vi "rs3 configure all 2.vi"(5 "Sensor in":u64, 11 "error in (no error)":errorcluster) -> (4 "config error":string, 6 "All Available streams":T1(array[cluster]), 8 "Sensor out":u64, 15 "error out":errorcluster)   [LabVIEW 2017, in "libRealSense3.lvlib"]
doc: "This VI configures the CAMERA-SENSOR to stream a specific set of 2 PROFILES.\n\nSteam selection: \nDepth+Left Color, \nUnrectified Left + Right (The raw input images)\nRectified Left + Right\n\nThe output array of STREAM PROFILE HANDLES is used to START the streams.\n\nThis VI also returns the BASELINE of the stereo module."
uses:
  libRealSense3.lvlib
panel:
  # "RS3 Configure All 2"
  # "(C) Intel Corp.,  AGJ 2017"
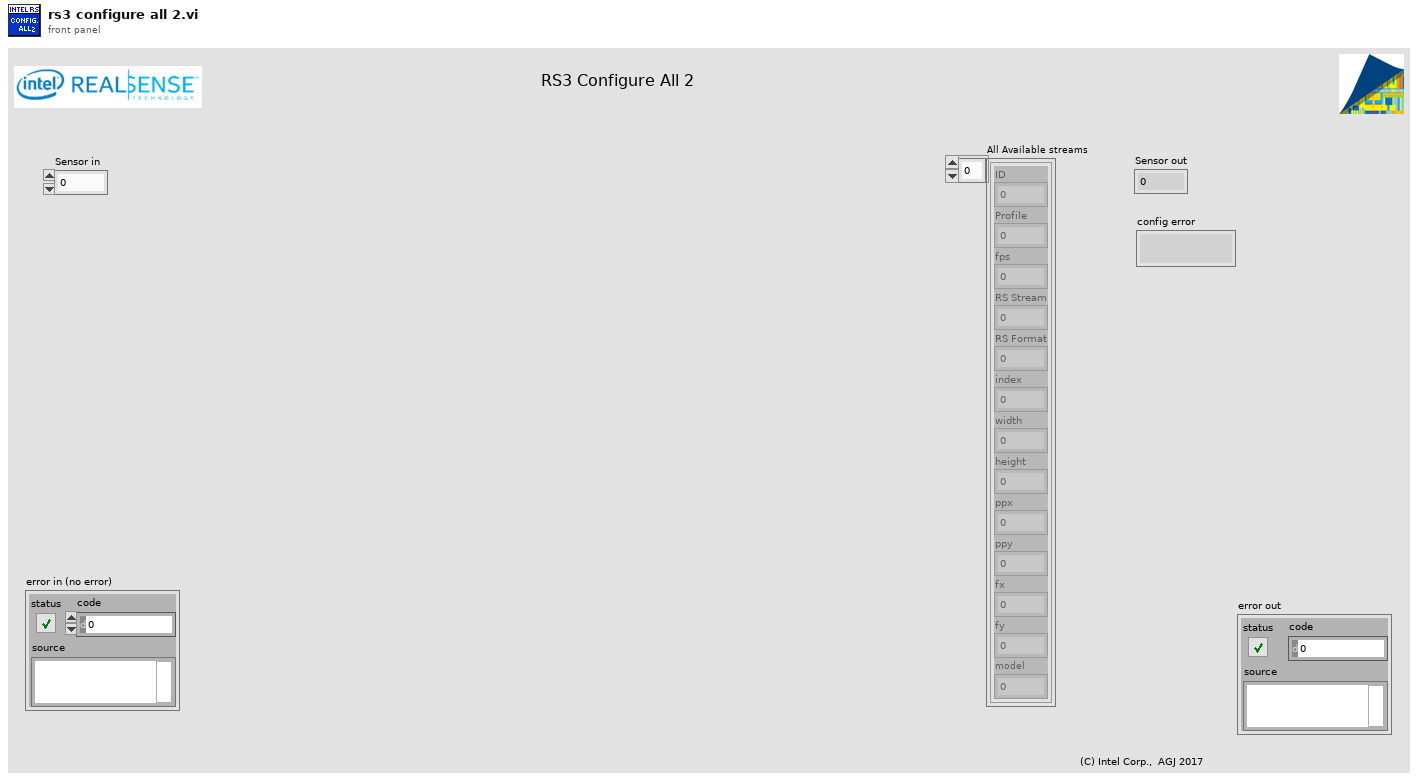
[diagram p1: front panel]
types:
  T1 = cluster{"ID":i32, "Profile":u64, "fps":i32, "RS Stream":u16, "RS Format":u16, "index":u16, "width":u16, "height":u16, "ppx":sgl, "ppy":sgl, "fx":sgl, "fy":sgl, "model":u32}[]
  T2 = cluster{"ID":i32, "Profile":u64, "fps":i32, "RS Stream":u16, "RS Format":u16, "index":u16, "width":u16, "height":u16, "ppx":sgl, "ppy":sgl, "fx":sgl, "fy":sgl, "model":u32}
  T3 = cluster{"width":i32, "height":i32, "ppx":sgl, "ppy":sgl, "fx":sgl, "fy":sgl, "model":u32, "coeffs[0]":sgl, "coeffs[1]":sgl, "coeffs[2]":sgl, "coeffs[3]":sgl, "coeffs[4]":sgl}
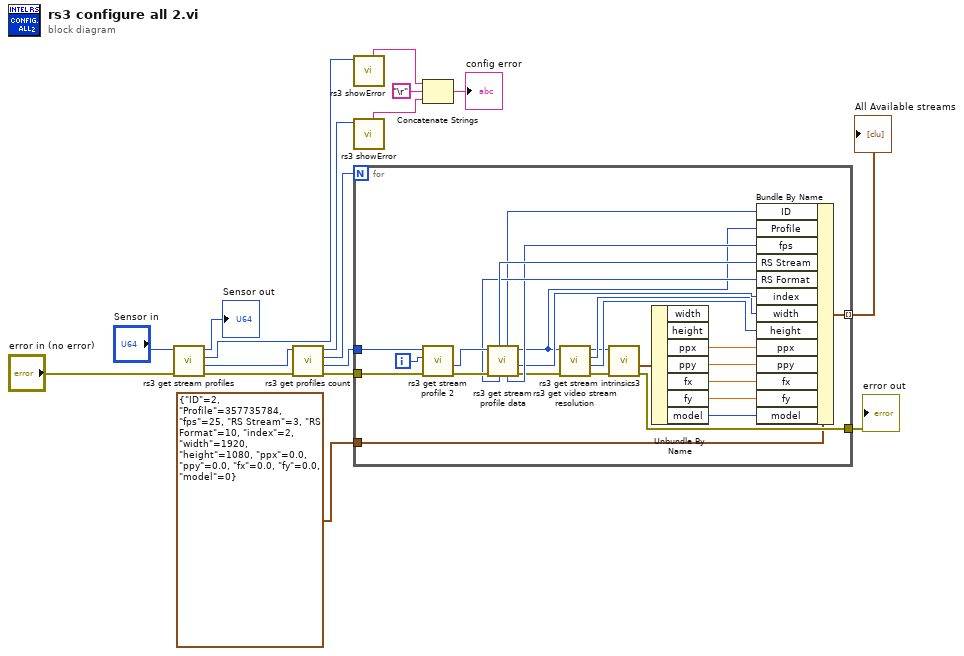
[diagram p0: block diagram]
diagram:
  n1 = call "rs3 get stream profiles.vi"("error in (no error)"="error in (no error)", "Sensor in"="Sensor in") -> (0:"error out"=w11:errorcluster, "Stream profile list"=w10:u64, 2:"error out"=w9:u64, "Sensor out"=→"Sensor out":u64)  [unwired: 6 in]
  n2 = call "rs3 get profiles count.vi"("error in"=w11, "Profiles_list"=w10) -> ("error out"=w13:errorcluster, "Profiles_list_out"=w14:u64, "Profiles count"=w15:i32, "error"=w12:u64)  [unwired: 6 in]
  n3 = call "rs3 showError.vi"("error"=w9) -> ("Error summary"=w7:string)  [unwired: 6 in, 4 out]
  n4 = call "rs3 showError.vi"("error"=w12) -> ("Error summary"=w5:string)  [unwired: 6 in, 4 out]
  n5 = for {
    N: w15 -> [_]
    tunnel: w13 -> [w42]
    tunnel: w14 -> [w41]
    tunnel: T2 {"ID"=2, "Profile"=357735784, "fps"=25, "RS Stream"=3, "RS Format"=10, "index"=2, "width"=1920, "height"=1080, "ppx"=0.0, "ppy"=0.0, "fx"=0.0, "fy"=0.0, "model"=0} ("output cluster") -> [w23]
    tunnel: [w32] -> w2 mode=indexing
    tunnel: [w25] -> w16
    i -> [w40]
    n6 = call "rs3 get stream profile 2.vi"("error in (no error)"=w42, "index"=w40, "Stream Profile list in"=w41) -> ("error out"=w38:errorcluster, "stream profile"=w39:u64)  [unwired: 5 in, 2 out]
    n7 = call "rs3 get stream profile data.vi"("error in (no error)"=w38, "Profile"=w39) -> ("error out"=w31:errorcluster, "index"=w33:i32, "Profile out"=w30:u64, "frame rate"=w35:i32, "unique id"=w34:i32, "RS Format"=w36:u16, "RS Stream"=w37:u16)  [unwired: 2 in, 1 out]
    n8 = call "rs3 get video stream resolution.vi"("error in (no error)"=w31, "Profile"=w30) -> ("error out"=w26:errorcluster, "height"=w29:u32, "width"=w28:u32, "Profile out"=w27:u64)  [unwired: 5 in, 1 out]
    n9 = call "rs3 get stream intrinsics3.vi"("error in (no error)"=w26, "stream profile"=w27) -> ("error out"=w25:errorcluster, "intrin out"=w24:T3)  [unwired: 6 in, 2 out]
    n10 = Unbundle By Name(w24) -> ("ppx"=w22:sgl, "ppy"=w21:sgl, "fx"=w20:sgl, "fy"=w19:sgl, "model"=w18:u32)  [unwired: 2 out]
    n11 = Bundle By Name(cluster=w23, "ID"=w34, "Profile"=w30, "fps"=w35, "RS Stream"=w37, "RS Format"=w36, "index"=w33, "width"=w28, "height"=w29, "ppx"=w22, "ppy"=w21, "fx"=w20, "fy"=w19, "model"=w18) -> (w32:T2)
  }
  "error out" <- w16
  "All Available streams" <- w2
  n12 = Concatenate Strings(w7, "\r", w5) -> (→"config error":string)
